vi "teleop template.vi"() -> ()   [LabVIEW 2018]
uses:
  <vilib>/Rock Robotics/WPI/DriverStation/WPI_DriverStationMatch Info.ctl
  <vilib>/Rock Robotics/WPI/DriverStation/WPI_DriverStationDerivedRobotMode.ctl
  <vilib>/Rock Robotics/WPI/Utilities/WPI_GetSetVariantRefNum.vi
  <vilib>/Rock Robotics/Network Tables/NT Write Numeric Array.vi
  <vilib>/Rock Robotics/Network Tables/NT Write Boolean.vi
  <vilib>/Rock Robotics/Network Tables/NT Read Boolean.vi
  <vilib>/Rock Robotics/Network Tables/NT Read Number.vi
panel:
  out "Sample Slider 1":dbl(slide) scale=0.0..5.0
  out "Sample Boolean 2":bool
  out "Sample Boolean 3":bool
  out "Sample Slider 0":dbl(slide) scale=0.0..5.0
  out "Sample Boolean 1":bool
  out "Sample Boolean 0":bool
  in  "Call Context":T1
  in  "Match Info":T2={"Autonomous Elapsed Seconds"=0.0, "TeleOp Elapsed Seconds"=0.0, "Disabled Elapsed Seconds"=0.0, "Visited Autonomous"=FALSE, "Visited TeleOp"=FALSE, "Visited Disabled"=FALSE, "Autonomous Settings"={"Autonomous Style"=enum."Independent", "VI Refnum"=refnum}}
  out "Left axis value":dbl
  out "Right axis value":dbl
  in  "Square Inputs":bool
  out "?":dbl
  out "?":dbl
  in  "Max Output":dbl=1.0 min=-1.0 max=1.0 step=0.1
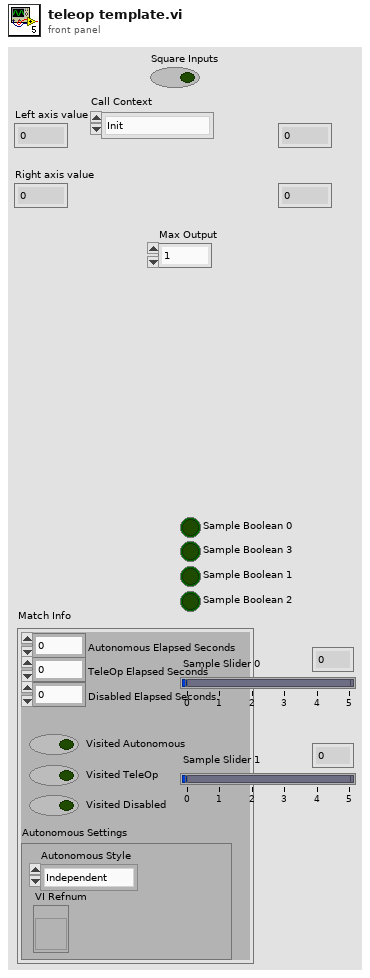
[diagram p1: front panel]
types:
  T1 = typedef "WPI_DriverStationDerivedRobotMode.ctl" = enum16{"Init", "Execute", "Stop"}
  T2 = typedef "WPI_DriverStationMatch Info.ctl" = cluster{"Autonomous Elapsed Seconds":dbl, "TeleOp Elapsed Seconds":dbl, "Disabled Elapsed Seconds":dbl, "Visited Autonomous":bool, "Visited TeleOp":bool, "Visited Disabled":bool, "Autonomous Settings":cluster{"Autonomous Style":enum16{"Iterative", "Independent"}, "VI Refnum":refnum<vi>}}
  T3 = typedef "WPI_JoystickDevRef.ctl" = cluster{"Device":T4}
  T4 = typedef "WPI_JoystickDeviceEnum.ctl" = enum16{"USB 0", "USB 1", "USB 2", "USB 3", "USB 4", "USB 5"}
  T5 = typedef "WPI_DigitalInputDevRef.ctl" = cluster{"DevStatus":errorcluster, "DIO Channel":T6}
  T6 = typedef "FPGA_DIOChannel.ctl" = enum8{"DIO 0", "DIO 1", "DIO 2", "DIO 3", "DIO 4", "DIO 5", "DIO 6", "DIO 7", "DIO 8", "DIO 9", "DIO MXP 0", "DIO MXP 1", "DIO MXP 2", "DIO MXP 3", "DIO MXP 4", "DIO MXP 5", "DIO MXP 6", "DIO MXP 7", "DIO MXP 8", "DIO MXP 9", "DIO MXP 10", "DIO MXP 11", "DIO MXP 12", "DIO MXP 13", "DIO MXP 14", "DIO MXP 15", "SPI Port CS1", "SPI Port CS2", "SPI Port CS3", "SPI Port MISO", "SPI Port MOSI", "Invalid"}
  T7 = typedef "WPI_MotorControlDeviceRef.ctl" = cluster{"DeviceStatus":errorcluster, "Type":T8, "PWM":cluster{"PWM Channel":T9, "DeadBand":T10}, "CAN":cluster{"Device Number":u8, "SetOutput VI Ref":variant, "GetOutput VI Ref":variant, "Enable VI Ref":variant, "Disable VI Ref":variant, "Data":variant}, "Invert":bool, "DIO PWM":cluster{"PWM \"Enable\" Channel":T9, "DIOChannel":T6, "PWM Rate":dbl}}
  T8 = typedef "WPI_MotorControlType.ctl" = enum16{"PWM", "CAN", "DIO PWM"}
  T9 = typedef "FPGA_DIOPWMChannel.ctl" = enum8{"PWM 0", "PWM 1", "PWM 2", "PWM 3", "PWM 4", "PWM 5", "PWM 6", "PWM 7", "PWM 8", "PWM 9", "PWM MXP 0", "PWM MXP 1", "PWM MXP 2", "PWM MXP 3", "PWM MXP 4", "PWM MXP 5", "PWM MXP 6", "PWM MXP 7", "PWM MXP 8", "PWM MXP 9", "Invalid"}
  T10 = typedef "WPI_PWMDeadband.ctl" = cluster{"Name":string, "maxPositivePwm":i32, "minPositivePwm":i32, "centerPwm":i32, "maxNegativePwm":i32, "minNegativePwm":i32, "angularRange":u16}
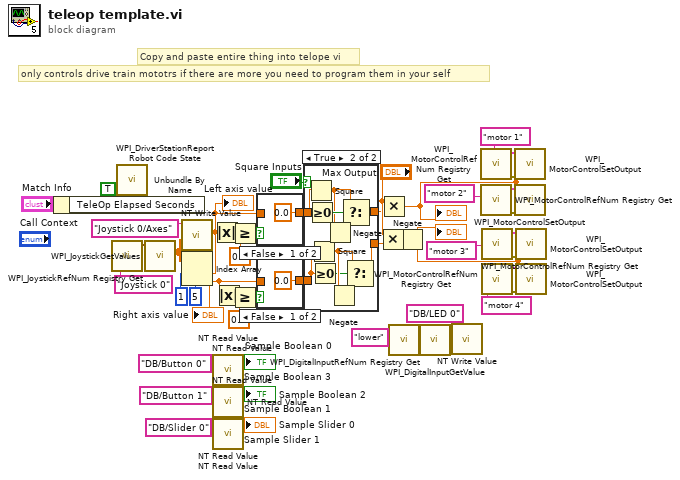
[diagram p0: block diagram]
diagram:
  # "only controls drive train mototrs if there are more you need to program them in your self"
  # "Copy and paste entire thing into telope vi"
  n1 = Unbundle By Name("Match Info") -> ()  [unwired: 1 out]
  n2 = call <vilib>:"WPI_JoystickRefNum Registry Get.vi"("refnum name"="Joystick 0") -> ("JoystickDevRef"=w53:T3)  [unwired: 1 in, 9 out]
  n3 = call <vilib>:"WPI_DriverStationReport Robot Code State.vi"("TeleOp"=TRUE ("Autonomous")) -> ()  [unwired: 10 in, 1 out]
  n4 = call <vilib>:"WPI_JoystickGetValues.vi"("JoystickDevRef"=w53) -> ("Axes"=w24:dbl[])  [unwired: 6 in, 4 out]
  n5 = call-poly <vilib>:"NT Write Value.vi"("Numeric Array"=w24, "Name"="Joystick 0/Axes") -> ()  [unwired: 9 in, 1 out]
  n6 = Index Array(array=w24, index #1=1 ("index"), index #2=5 ("index")) -> (element #1=w17:dbl, element #2=w16:dbl)
  "Right axis value" <- w16
  "Left axis value" <- w17
  n7 = Absolute Value(x=w17) -> (abs(x)=w29:dbl)
  n8 = call-poly <vilib>:"NT Read Value.vi"("Name"="DB/Button 0" ("refnum name")) -> ("Boolean"=→"Sample Boolean 3":bool)  [unwired: 9 in, 1 out]
  n9 = call-poly <vilib>:"NT Read Value.vi"("Name"="DB/Button 0" ("refnum name")) -> ("Boolean"=→"Sample Boolean 0":bool)  [unwired: 9 in, 1 out]
  n10 = call-poly <vilib>:"NT Read Value.vi"("Name"="DB/Button 1" ("refnum name")) -> ("Boolean"=→"Sample Boolean 2":bool)  [unwired: 9 in, 1 out]
  n11 = call-poly <vilib>:"NT Read Value.vi"("Name"="DB/Button 1" ("refnum name")) -> ("Boolean"=→"Sample Boolean 1":bool)  [unwired: 9 in, 1 out]
  n12 = call-poly <vilib>:"NT Read Value.vi"("Name"="DB/Slider 0" ("refnum name")) -> ("Numeric"=→"Sample Slider 1":dbl)  [unwired: 9 in, 1 out]
  n13 = call-poly <vilib>:"NT Read Value.vi"("Name"="DB/Slider 0" ("refnum name")) -> ("Numeric"=→"Sample Slider 0":dbl)  [unwired: 9 in, 1 out]
  n14 = Absolute Value(x=w16) -> (abs(x)=w28:dbl)
  n15 = Greater Or Equal?(x=w29, y=0.2) -> (x >= y?=w30:bool)
  n16 = Greater Or Equal?(x=w28, y=0.2) -> (x >= y?=w27:bool)
  n17 = case shown="False" w30 {
    tunnel: [0.0 ("upper limit") w56] -> w18
    tunnel: w17 -> [_ w56]
    frame False {
    }
    frame True {
    }
  }
  n18 = case shown="False" w27 {
    tunnel: [0.0 ("upper limit") w58] -> w25
    tunnel: w16 -> [_ w58]
    frame False {
    }
    frame True {
    }
  }
  n19 = case shown="True" "Square Inputs" {
    tunnel: w18 -> [w60 w70]
    tunnel: [w60 w66] -> w45
    tunnel: [w59 w62] -> w47
    tunnel: w25 -> [w59 w61]
    frame False {
    }
    frame True {
      n20 = Square(x=w70) -> (x^2=w68:dbl)
      n21 = Greater Or Equal To 0?(x=w70) -> (x >= 0?=w69:bool)
      n22 = Square(x=w61) -> (x^2=w64:dbl)
      n23 = Greater Or Equal To 0?(x=w61) -> (x >= 0?=w63:bool)
      n24 = Negate(x=w68) -> (-x=w67:dbl)
      n25 = Negate(x=w64) -> (-x=w65:dbl)
      n26 = Select(t=w68, s=w69, f=w67) -> (s? t:f=w66:dbl)
      n27 = Select(t=w64, s=w63, f=w65) -> (s? t:f=w62:dbl)
    }
  }
  n28 = Multiply(x="Max Output", y=w47) -> (x*y=w32:dbl)
  n29 = Multiply(x="Max Output", y=w45) -> (x*y=w15:dbl)
  "?" <- w15
  n30 = call <vilib>:"WPI_DigitalInputRefNum Registry Get.vi"("refnum name"="lower") -> ("error out"=w22:errorcluster, "DigitalInputDevRef"=w21:T5)  [unwired: 9 in]
  n31 = Negate(x=w32) -> (-x=w33:dbl)
  "?" <- w33
  n32 = call <vilib>:"WPI_DigitalInputGetValue.vi"("error in (no error)"=w22, "DigitalInputDevRef"=w21) -> ("Value"=w19:bool)  [unwired: 7 in, 2 out]
  n33 = call-poly <vilib>:"NT Write Value.vi"("Boolean"=w19, "Name"="DB/LED 0") -> ()  [unwired: 9 in, 1 out]
  n34 = call <vilib>:"WPI_MotorControlRefNum Registry Get.vi"("refnum name"="motor 1") -> ("error out"=w50:errorcluster, "MotorControlDevRef"=w49:T7)  [unwired: 9 in]
  n35 = call <vilib>:"WPI_MotorControlRefNum Registry Get.vi"("refnum name"="motor 2") -> ("error out"=w41:errorcluster, "MotorControlDevRef"=w42:T7)  [unwired: 9 in]
  n36 = call <vilib>:"WPI_MotorControlRefNum Registry Get.vi"("refnum name"="motor 3") -> ("error out"=w38:errorcluster, "MotorControlDevRef"=w37:T7)  [unwired: 9 in]
  n37 = call <vilib>:"WPI_MotorControlRefNum Registry Get.vi"("refnum name"="motor 4") -> ("error out"=w35:errorcluster, "MotorControlDevRef"=w36:T7)  [unwired: 9 in]
  n38 = call <vilib>:"WPI_MotorControlSetOutput.vi"("error in (no error)"=w50, "Output"=w15, "MotorControlDevRef"=w49) -> ()  [unwired: 6 in, 3 out]
  n39 = call <vilib>:"WPI_MotorControlSetOutput.vi"("error in (no error)"=w41, "Output"=w15, "MotorControlDevRef"=w42) -> ()  [unwired: 6 in, 3 out]
  n40 = call <vilib>:"WPI_MotorControlSetOutput.vi"("error in (no error)"=w38, "Output"=w33, "MotorControlDevRef"=w37) -> ()  [unwired: 6 in, 3 out]
  n41 = call <vilib>:"WPI_MotorControlSetOutput.vi"("error in (no error)"=w35, "Output"=w33, "MotorControlDevRef"=w36) -> ()  [unwired: 6 in, 3 out]
